vi "EXE FWLoader.vi"() -> ()   [LabVIEW 2010, in "lib1299.lvlib"]
uses:
  lib1299.lvlib
  Controls/FW State.ctl
panel:
  out "FW Load Debug":T1
  out "Overall Progress":u8(slide) scale=0.0..7.0
  in  "Firmware file":path
  out "Status box":string
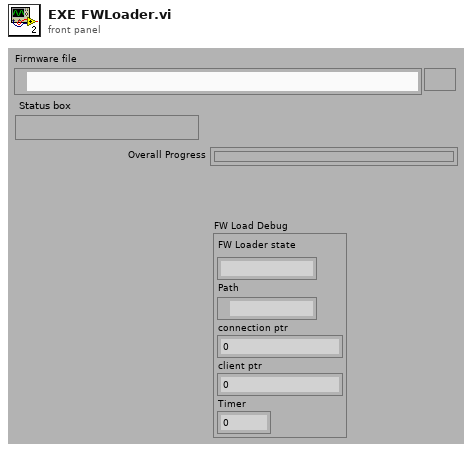
[diagram p1: front panel]
types:
  T1 = typedef "lib1299.lvlib/FW State.ctl" = cluster{"FW Loader state":string, "Path":path, "connection ptr":i32, "client ptr":i32, "Timer":i64}
  T2 = enum32{"invalid app kind", "Development System", "Run Time System", "Student Edition", "Embedded LabVIEW", "Evaluation", "Custom"}
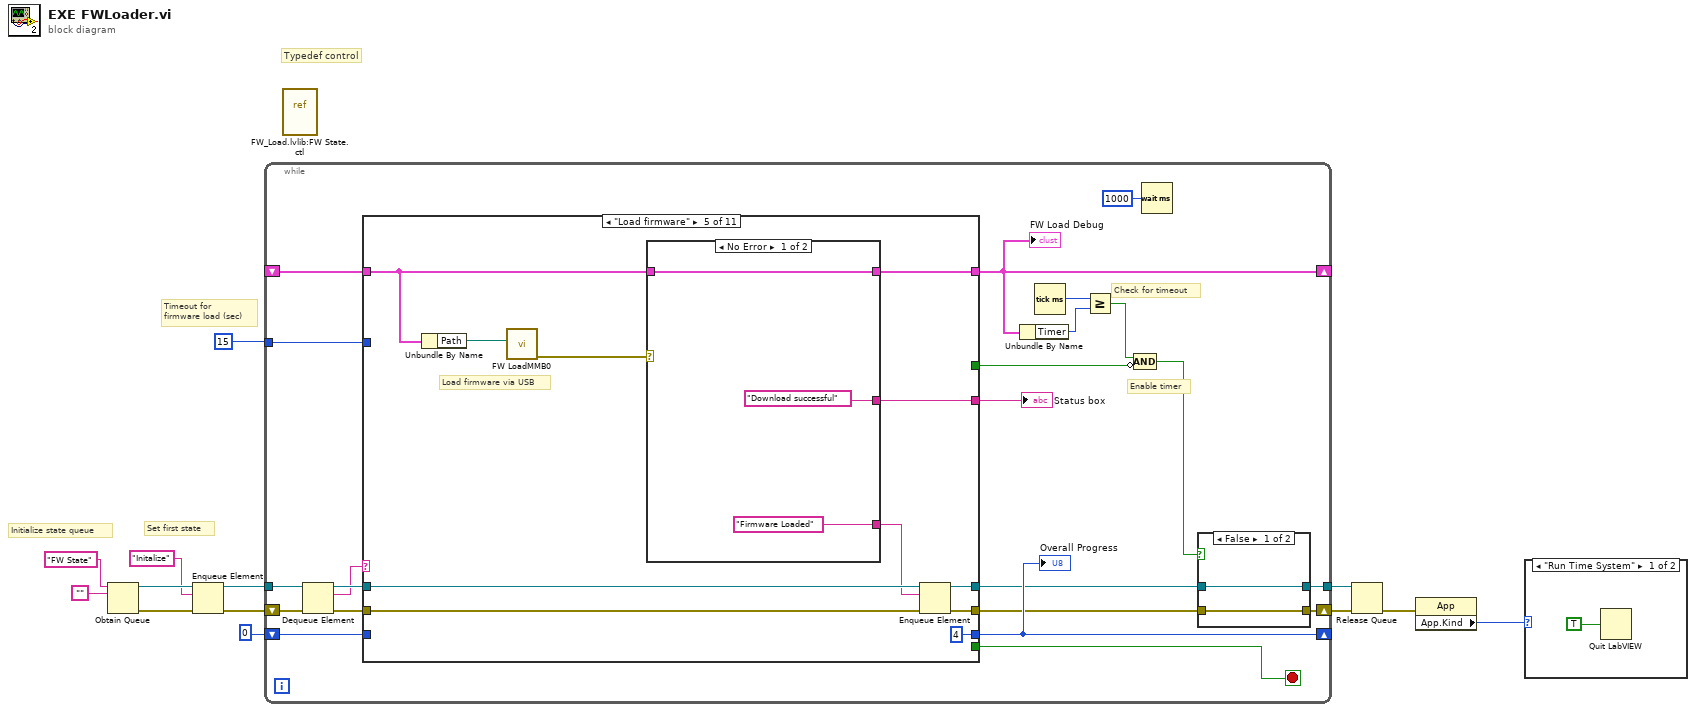
[diagram p0: block diagram]
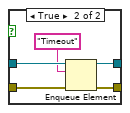
[diagram p3: hidden frame]
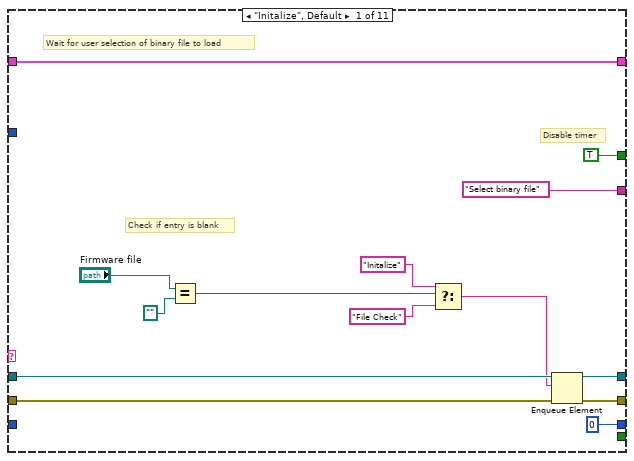
[diagram p4: hidden frame]
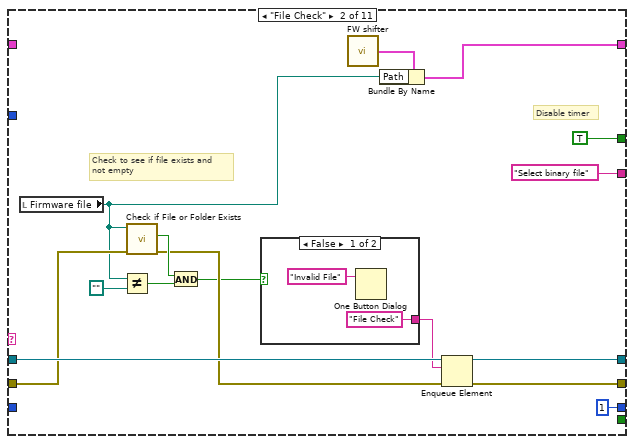
[diagram p5: hidden frame]
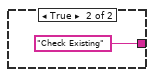
[diagram p6: hidden frame]
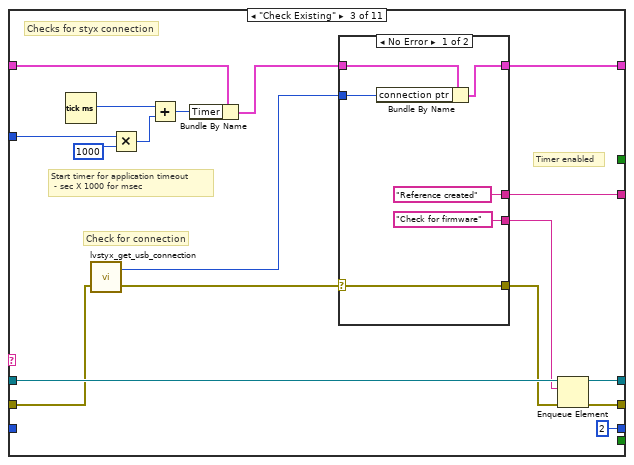
[diagram p7: hidden frame]
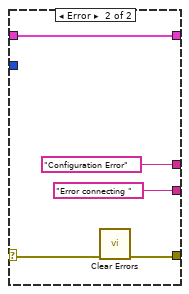
[diagram p8: hidden frame]
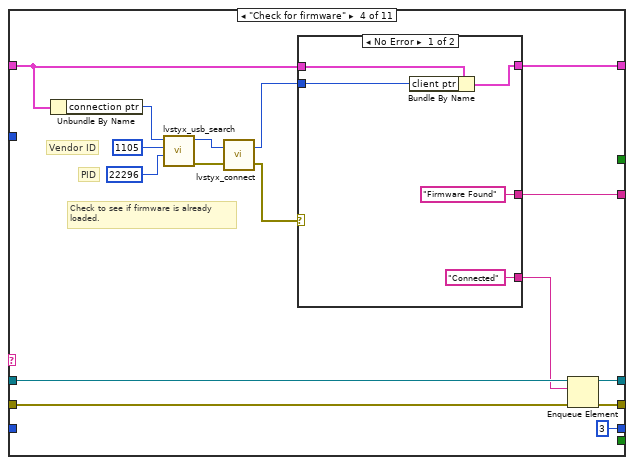
[diagram p9: hidden frame]
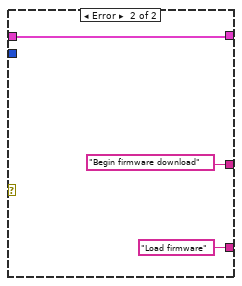
[diagram p10: hidden frame]
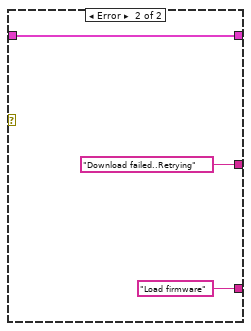
[diagram p11: hidden frame]
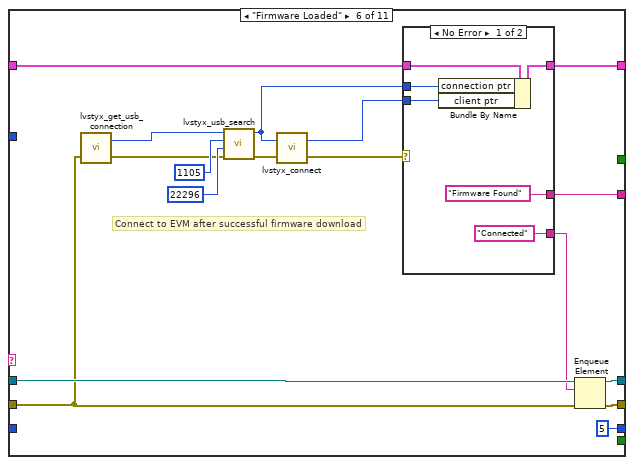
[diagram p12: hidden frame]
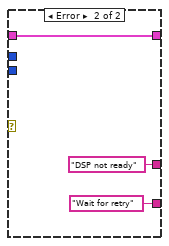
[diagram p13: hidden frame]
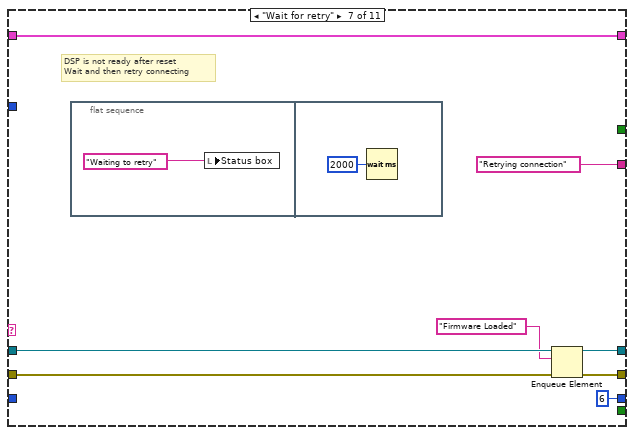
[diagram p14: hidden frame]
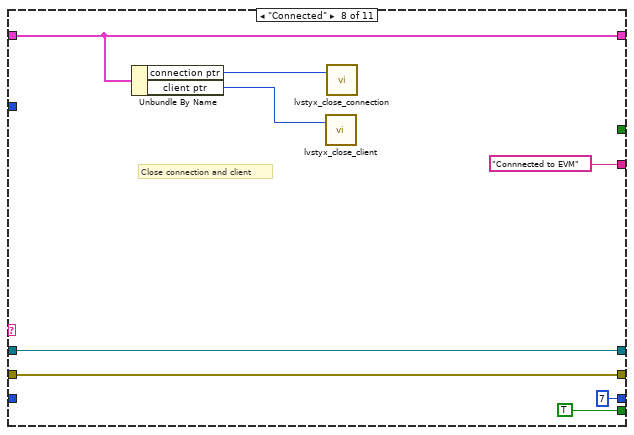
[diagram p15: hidden frame]
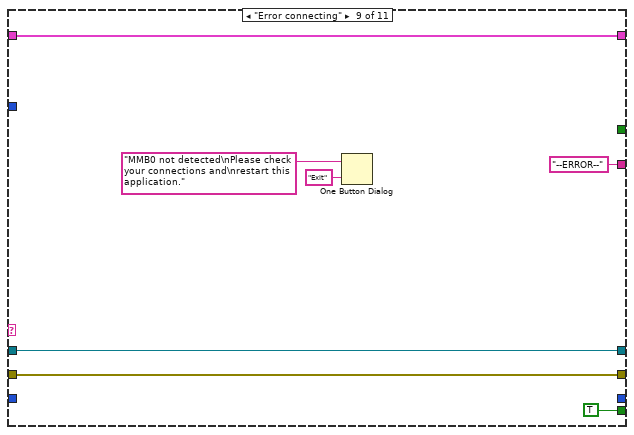
[diagram p16: hidden frame]
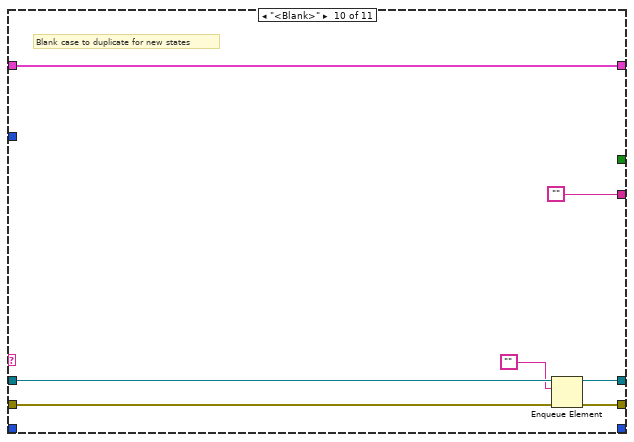
[diagram p17: hidden frame]
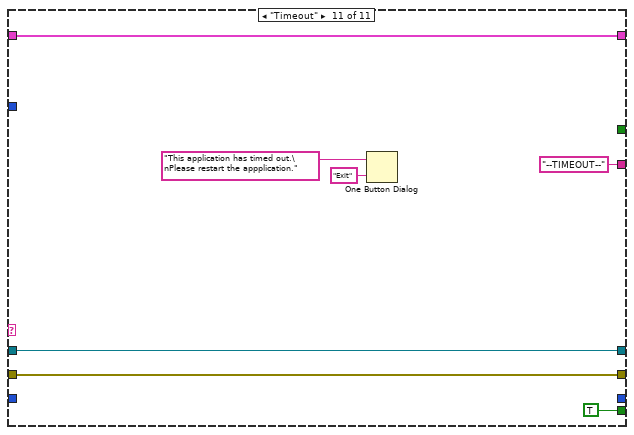
[diagram p18: hidden frame]
diagram:
  # "Typedef control"
  # "Set first state"
  # "Initialize state queue"
  # "Timeout for\nfirmware load (sec)"
  n1 = Obtain Queue(name (unnamed)="FW State", element data type="") -> (queue out=w13:refnum<queue>, error out=w12:errorcluster)  [unwired: 3 in, 1 out]
  n2 = Enqueue Element(queue=w13, element="Initalize", error in (no error)=w12) -> (queue out=w11:refnum<queue>, error out=w7:errorcluster)  [unwired: 1 in, 1 out]
  n3 = while {
    shift-right: [w27] -> _
    shift-left: _ -> [w29]
    shift-right: [w15] -> w6
    shift-left: w7 -> [w30]
    tunnel: 15 ("y") -> [w26]
    shift-right: [w20] -> _
    shift-left: 0 -> [w21]
    tunnel: w11 -> [w35]
    tunnel: [w16] -> w5
    stop <- w19 stop-if-true
    # "Enable timer"
    # "Check for timeout"
    n4 = Dequeue Element(queue=w35, error in (no error)=w30) -> (queue out=w34:refnum<queue>, element=w33:string, error out=w32:errorcluster)  [unwired: 1 in, 1 out]
    n5 = case shown="\"Load firmware\"" w33 {
      tunnel: w34 -> [w54 w69 w91 w118 w137 w160 w177 w189 w193 w201 w209]
      tunnel: w32 -> [w53 w65 w90 w117 w136 w155 w176 w188 w192 w200 w208]
      tunnel: [w56 w68 w93 w120 w139 w162 w179 w189 w193 w203 w209] -> w18
      tunnel: [w52 w66 w86 w107 w131 w149 w175 w185 w196 w197 w210] -> w27
      tunnel: [w55 w61 w92 w119 w138 w161 w178 w188 w192 w202 w208] -> w17
      tunnel: w29 -> [w52 _ w79 w108 w130 w150 w175 w185 w196 w197 w210]
      tunnel: ["Select binary file" "Select binary file" w84 w109 w133 w148 "Retrying connection" "Connnected to EVM" "--ERROR--" "" "--TIMEOUT--"] -> w28
      tunnel: [_ _ _ _ _ _ _ TRUE TRUE _ TRUE] -> w19
      tunnel: w26 -> [_ _ w80 _ _ _ _ _ _ _ _]
      tunnel: [TRUE TRUE _ _ _ _ _ _ _ _ _] -> w23
      tunnel: w21 -> [_ _ _ _ _ _ _ _ _ _ _]
      tunnel: [0 1 2 3 4 5 6 7 _ _ _] -> w20
      frame "Initalize", Default {
        # "Disable timer"
        # "Check if entry is blank"
        # "Wait for user selection of binary file to load"
        n6 = Equal?(x="Firmware file", y=path "") -> (x = y?=w46:bool)
        n7 = Select(t="Initalize", s=w46, f="File Check") -> (s? t:f=w48:string)
        n8 = Enqueue Element(queue=w54, element=w48, error in (no error)=w53) -> (queue out=w56:refnum<queue>, error out=w55:errorcluster)  [unwired: 1 in, 1 out]
      }
      frame "File Check" {
        # "Check to see if file exists and\nnot empty"
        # "Disable timer"
        n9 = local read "Firmware file"() -> (w58:path)
        n10 = Not Equal?(x=w58, y=path "") -> (x != y?=w72:bool)
        n11 = call <vilib>:"Check if File or Folder Exists.vi"("error in (no error)"=w65, "path"=w58) -> ("error out"=w64:errorcluster, "file or folder exists?"=w71:bool)  [unwired: 7 in, 1 out]
        n12 = And(x=w71, y=w72) -> (x .and. y?=w63:bool)
        n13 = case shown="False" w63 {
          tunnel: ["File Check" "Check Existing"] -> w62
          frame False {
            n14 = One Button Dialog(message="Invalid File") -> ()  [unwired: 1 in, 1 out]
          }
          frame True {
          }
        }
        n15 = call "FW shifter.vi"() -> ("Cluster"=w67:T1)  [unwired: 1 in]
        n16 = Bundle By Name(cluster=w67, "Path"=w58) -> (w66:T1)
        n17 = Enqueue Element(queue=w69, element=w62, error in (no error)=w64) -> (queue out=w68:refnum<queue>, error out=w61:errorcluster)  [unwired: 1 in, 1 out]
      }
      frame "Check Existing" {
        # "Timer enabled"
        # "Checks for styx connection"
        # "Check for connection"
        # "Start timer for application timeout\n - sec X 1000 for msec"
        n18 = Tick Count (ms)() -> (millisecond timer value=w82:u32)
        n19 = call "lvstyx_get_usb_connection.vi"("error in (no error)"=w90) -> ("error out"=w89:errorcluster, "connection ptr"=w85:u32)  [unwired: 1 in]
        n20 = Multiply(x=w80, y=1000) -> (x*y=w83:i32)
        n21 = Add(x=w82, y=w83) -> (x+y=w77:u32)
        n22 = Bundle By Name(cluster=w79, "Timer"=w77) -> (w78:T1)
        n23 = case shown="No Error" w89 {
          selector: w89 -> [w99 w103]
          tunnel: [w99 w104] -> w88
          tunnel: ["Check for firmware" "Error connecting "] -> w87
          tunnel: w78 -> [w95 w100]
          tunnel: [w94 w100] -> w86
          tunnel: w85 -> [w96 _]
          tunnel: ["Reference created" "Configuration Error"] -> w84
          frame No Error {
            n24 = Bundle By Name(cluster=w95, "connection ptr"=w96) -> (w94:T1)
          }
          frame Error {
            n25 = call <vilib>:"Clear Errors.vi"("error in (no error)"=w103) -> ("error out"=w104:errorcluster)  [unwired: 6 in]
          }
        }
        n26 = Enqueue Element(queue=w91, element=w87, error in (no error)=w88) -> (queue out=w93:refnum<queue>, error out=w92:errorcluster)  [unwired: 1 in, 1 out]
      }
      frame "Check for firmware" {
        # "PID"
        # "Vendor ID"
        # "Check to see if firmware is already\nloaded."
        n27 = Unbundle By Name(w108) -> ("connection ptr"=w113:i32)
        n28 = call "lvstyx_usb_search.vi"("pid"=u16 22296, "vid"=u16 1105, "conn ptr"=w113) -> ("error out"=w115:errorcluster, "dup conn ptr"=w111:u32)  [unwired: 6 in, 1 out]
        n29 = call "lvstyx_connect.vi"("error in (no error)"=w115, "connection ptr"=w111) -> ("error out"=w112:errorcluster, "client ptr"=w106:u32)
        n30 = case shown="No Error" w112 {
          tunnel: ["Connected" "Load firmware"] -> w110
          tunnel: ["Firmware Found" "Begin firmware download"] -> w109
          tunnel: w108 -> [w123 w126]
          tunnel: [w122 w126] -> w107
          tunnel: w106 -> [w121 _]
          frame No Error {
            n31 = Bundle By Name(cluster=w123, "client ptr"=w121) -> (w122:T1)
          }
          frame Error {
          }
        }
        n32 = Enqueue Element(queue=w118, element=w110, error in (no error)=w117) -> (queue out=w120:refnum<queue>, error out=w119:errorcluster)  [unwired: 1 in, 1 out]
      }
      frame "Load firmware" {
        # "Load firmware via USB"
        n33 = Unbundle By Name(w130) -> ("Path"=w135:path)
        n34 = call "FW LoadMMB0.vi"("Boot file"=w135) -> ("error out"=w134:errorcluster)  [unwired: 10 in]
        n35 = case shown="No Error" w134 {
          tunnel: ["Download successful" "Download failed..Retrying"] -> w133
          tunnel: ["Firmware Loaded" "Load firmware"] -> w132
          tunnel: [w140 w145] -> w131
          tunnel: w130 -> [w140 w145]
          frame No Error {
          }
          frame Error {
          }
        }
        n36 = Enqueue Element(queue=w137, element=w132, error in (no error)=w136) -> (queue out=w139:refnum<queue>, error out=w138:errorcluster)  [unwired: 1 in, 1 out]
      }
      frame "Firmware Loaded" {
        # "Connect to EVM after successful firmware download"
        n37 = call "lvstyx_get_usb_connection.vi"("error in (no error)"=w155) -> ("error out"=w154:errorcluster, "connection ptr"=w156:u32)  [unwired: 1 in]
        n38 = call "lvstyx_usb_search.vi"("error in (no error)"=w154, "pid"=u16 22296, "vid"=u16 1105, "conn ptr"=w156) -> ("error out"=w157:errorcluster, "dup conn ptr"=w151:u32)  [unwired: 5 in, 1 out]
        n39 = call "lvstyx_connect.vi"("error in (no error)"=w157, "connection ptr"=w151) -> ("error out"=w153:errorcluster, "client ptr"=w152:u32)
        n40 = case shown="No Error" w153 {
          tunnel: w152 -> [w165 _]
          tunnel: w151 -> [w166 _]
          tunnel: w150 -> [w168 w171]
          tunnel: [w167 w171] -> w149
          tunnel: ["Firmware Found" "DSP not ready"] -> w148
          tunnel: ["Connected" "Wait for retry"] -> w147
          frame No Error {
            n41 = Bundle By Name(cluster=w168, "connection ptr"=w166, "client ptr"=w165) -> (w167:T1)
          }
          frame Error {
          }
        }
        n42 = Enqueue Element(queue=w160, element=w147, error in (no error)=w155) -> (queue out=w162:refnum<queue>, error out=w161:errorcluster)  [unwired: 1 in, 1 out]
      }
      frame "Wait for retry" {
        # "DSP is not ready after reset\nWait and then retry connecting"
        n43 = flat-sequence {
          frame #0 {
            n44 = local write "Status box"("Waiting to retry") -> ()
          }
          frame #1 {
            n45 = Wait (ms)(milliseconds to wait=u32 2000) -> ()  [unwired: 1 out]
          }
        }
        n46 = Enqueue Element(queue=w177, element="Firmware Loaded", error in (no error)=w176) -> (queue out=w179:refnum<queue>, error out=w178:errorcluster)  [unwired: 1 in, 1 out]
      }
      frame "Connected" {
        # "Close connection and client"
        n47 = Unbundle By Name(w185) -> ("connection ptr"=w184:i32, "client ptr"=w183:i32)
        n48 = call "lvstyx_close_client.vi"("client ptr"=w183) -> ()  [unwired: 2 in, 1 out]
        n49 = call "lvstyx_close_connection.vi"("connection ptr"=w184) -> ()  [unwired: 2 in, 1 out]
      }
      frame "Error connecting" {
        n50 = One Button Dialog(message="MMB0 not detected\nPlease check your connections and\nrestart this application.", button name ("OK")="Exit") -> ()  [unwired: 1 out]
      }
      frame "<Blank>" {
        # "Blank case to duplicate for new states"
        n51 = Enqueue Element(queue=w201, element="", error in (no error)=w200) -> (queue out=w203:refnum<queue>, error out=w202:errorcluster)  [unwired: 1 in, 1 out]
      }
      frame "Timeout" {
        n52 = One Button Dialog(message="This application has timed out.\nPlease restart the appplication.", button name ("OK")="Exit") -> ()  [unwired: 1 out]
      }
    }
    "Status box" <- w28
    "Overall Progress" <- w20
    "FW Load Debug" <- w27
    n53 = Unbundle By Name(w27) -> ("Timer"=w24:i64)
    n54 = Tick Count (ms)() -> (millisecond timer value=w25:u32)
    n55 = Greater Or Equal?(x=w25, y=w24) -> (x >= y?=w22:bool)
    n56 = Compound Arithmetic op=AND(w22, invert w23) -> (w14:bool)
    n57 = Wait (ms)(milliseconds to wait=u32 1000) -> ()  [unwired: 1 out]
    n58 = case shown="False" w14 {
      tunnel: w18 -> [w37 w42]
      tunnel: w17 -> [w36 w41]
      tunnel: [w37 w40] -> w16
      tunnel: [w36 w39] -> w15
      frame False {
      }
      frame True {
        n59 = Enqueue Element(queue=w42, element="Timeout", error in (no error)=w41) -> (queue out=w40:refnum<queue>, error out=w39:errorcluster)  [unwired: 1 in, 1 out]
      }
    }
  }
  n60 = vi-ref "FW_Load.lvlib:FW State.ctl"() -> ()  [unwired: 1 out]
  n61 = Release Queue(queue=w5, error in (no error)=w6) -> (error out=w1:errorcluster)  [unwired: 1 in, 2 out]
  n62 = property class="App"(error in=w1) -> ("App.Kind"=w2:T2)  [unwired: 1 in, 2 out]
  n63 = case shown="\"Run Time System\"" w2 {
    frame "Run Time System" {
      n64 = Quit LabVIEW(quit? (T)=TRUE) -> ()
    }
    frame "Development System", Default {
    }
  }
